vi "LabVIEW IV 2주차.vi"() -> ()   [LabVIEW 2025]
uses:
  <vilib>/Analysis/1siggen.llb/Ramp Pattern by Samples.vi
  <vilib>/Analysis/NI_AALBase.lvlib
panel:
  in  "VISA resource name 2":refnum<visa-resource-name>
  in  "Start":bool
  in  "Both forward & backward sweep":bool=TRUE
  in  "VISA resource name":refnum<visa-resource-name>="GPIB0::15::INSTR"
  in  "stop":bool
  in  "samples":i32=128
  in  "Voltage End":dbl=1.0
  in  "Voltage start":dbl
  out "XY Graph":cluster{"Y":dbl[], "Y":dbl[]}[](graph)
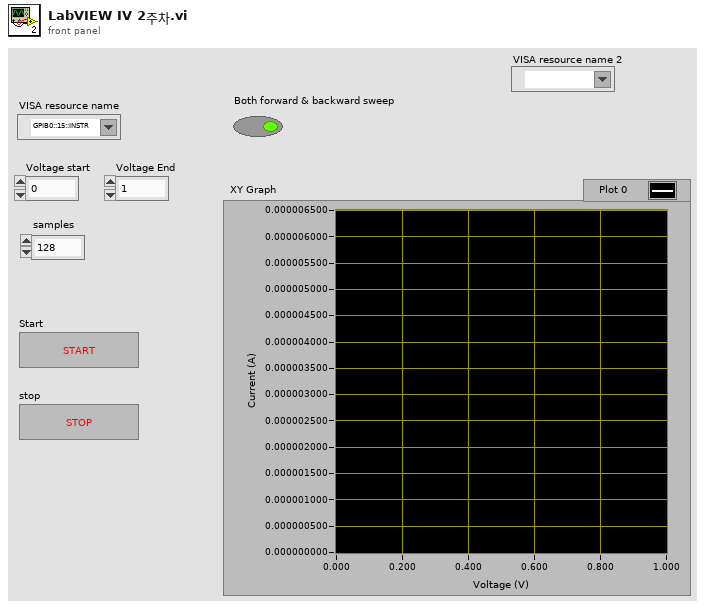
[diagram p1: front panel]
types:
  T1 = enum16{"open", "replace", "create", "open or create", "replace or create", "replace or create with confirmation"}
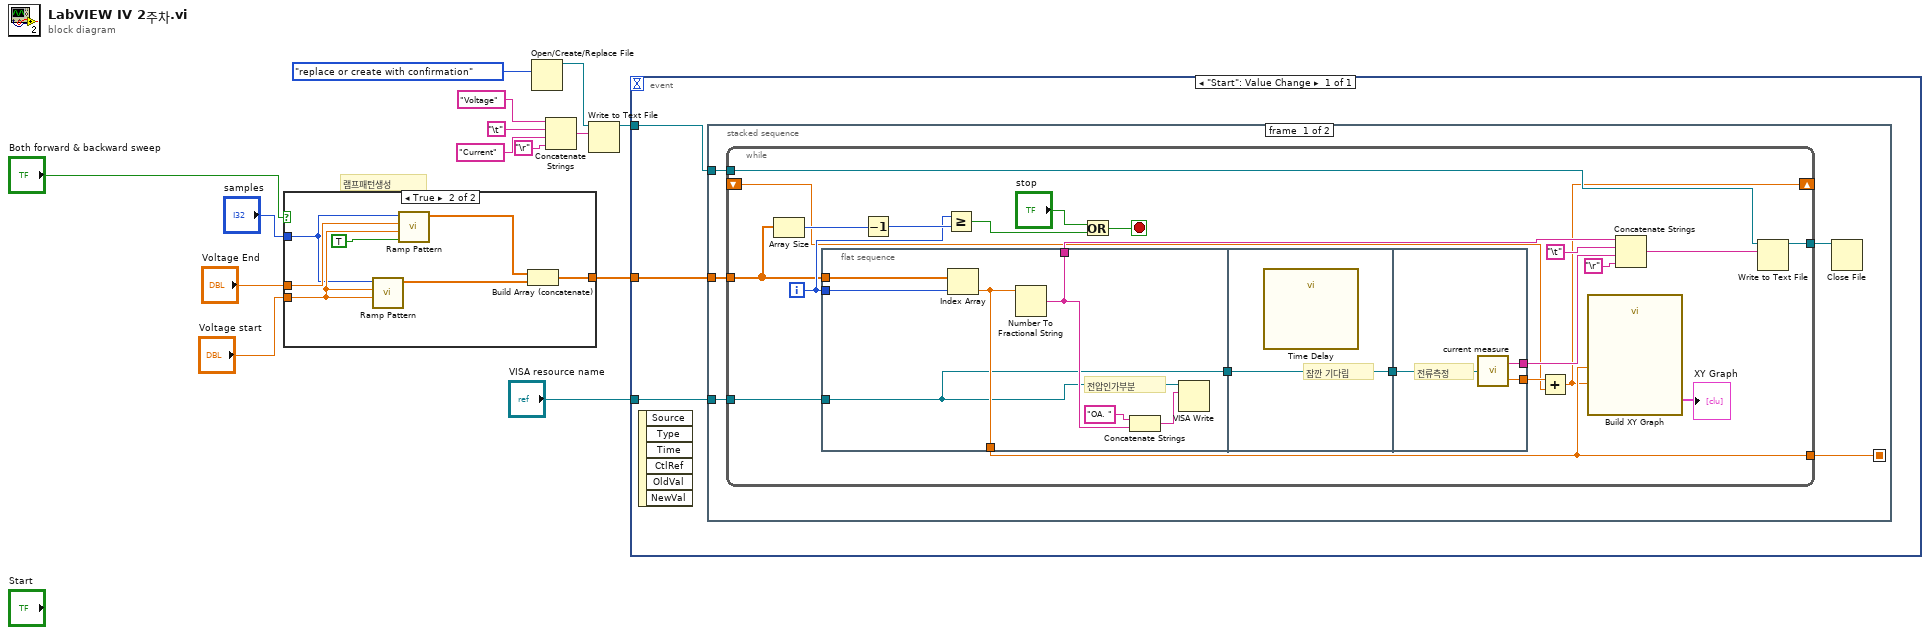
[diagram p0: block diagram]
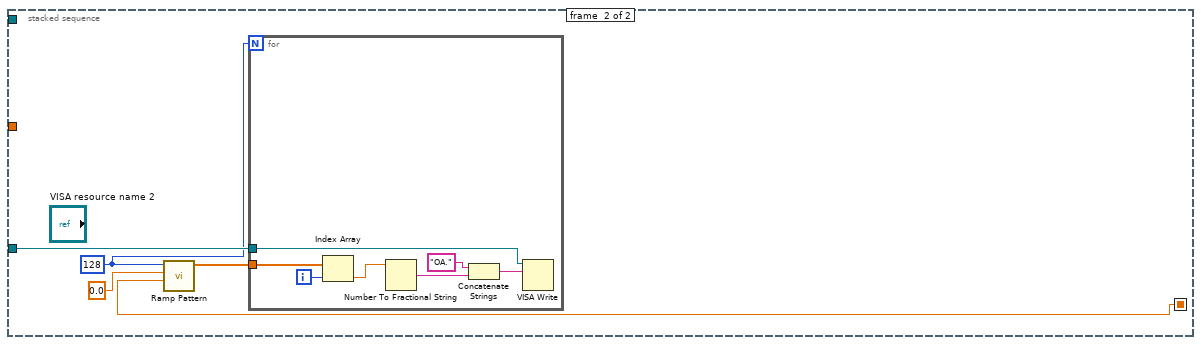
[diagram p2: hidden frame]
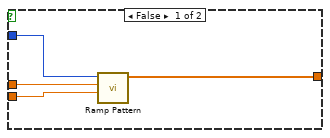
[diagram p3: hidden frame]
diagram:
  # "램프패턴생성"
  n1 = case shown="True" "Both forward & backward sweep" {
    tunnel: "Voltage start" -> [w18 w24]
    tunnel: "Voltage End" -> [w17 w25]
    tunnel: [w16 w19] -> w12
    tunnel: "samples" -> [w15 w23]
    frame False {
      n2 = call-poly <vilib>:"Ramp Pattern.vi"("start"=w18, "end"=w17, "samples"=w15) -> ("Ramp Pattern"=w16:dbl[])  [unwired: 7 in, 1 out]
    }
    frame True {
      n3 = call-poly <vilib>:"Ramp Pattern.vi"("start"=w24, "end"=w24, "samples"=w23) -> ("Ramp Pattern"=w20:dbl[])  [unwired: 7 in, 1 out]
      n4 = call-poly <vilib>:"Ramp Pattern.vi"("exclude end?"=TRUE, "start"=w24, "end"=w25, "samples"=w23) -> ("Ramp Pattern"=w21:dbl[])  [unwired: 6 in, 1 out]
      n5 = Build Array (concatenate)(w21, w20) -> (w19:dbl[])
    }
  }
  n6 = Open/Create/Replace File(operation (0:open)=T1."replace or create with confirmation") -> (refnum out=w9:refnum<file>)  [unwired: 5 in, 2 out]
  n7 = Concatenate Strings("Voltage" ("string"), "\t", "Current" ("string"), "\r") -> (w6:string)
  n8 = Write to Text File(file (use dialog)=w9, text=w6) -> (refnum out=w3:refnum<file>)  [unwired: 2 in, 2 out]
  n9 = event shown="[0] \"Start\": Value Change" {
    selector: _ -> [_]
    dyn-events: _ -> [_]
    timeout: _ -> [_]
    tunnel: w12 -> [w28]
    tunnel: w3 -> [w27]
    tunnel: "VISA resource name" -> [w26]
    event "Start": Value Change {
      n10 = event-data() -> ()  [unwired: 1 in, 6 out]
      n11 = stacked-sequence {
        seq-local: [w29 _] -> [_ w70]
        tunnel: w28 -> [w33 _]
        tunnel: w27 -> [w31 _]
        tunnel: w26 -> [w30 w68]
        frame #0 {
          n12 = while {
            tunnel: w33 -> [w40]
            tunnel: w31 -> [w50]
            tunnel: [w49] -> w32
            tunnel: w30 -> [w43]
            tunnel: [w37] -> w29
            shift-right: [w34] -> _
            shift-left: _ -> [w35]
            i -> [w51]
            stop <- w38 stop-if-true
            n13 = Array Size(array=w40) -> (size(s)=w39:i32)
            n14 = flat-sequence {
              tunnel: w40 -> [w62]
              tunnel: w51 -> [w61]
              tunnel: [w60] -> w37
              tunnel: [w57] -> w48
              tunnel: w43 -> [w56]
              tunnel: [w56] -> w41
              tunnel: [w63] -> w42
              tunnel: w41 -> [w63]
              tunnel: [w65] -> w47
              tunnel: w42 -> [w66]
              tunnel: [w64] -> w36
              frame #0 {
                # "전압인가부분"
                n15 = Index Array(array=w62, index=w61) -> (element=w60:dbl)
                n16 = Number To Fractional String(number=w60) -> (F-format string=w57:string)  [unwired: 3 in]
                n17 = Concatenate Strings("OA. " ("write buffer"), w57) -> (w59:string)
                n18 = VISA Write(VISA resource name=w56, write buffer=w59) -> ()  [unwired: 1 in, 3 out]
              }
              frame #1 {
                # "잠깐 기다림"
                n19 = call "Time Delay"() -> ()  [unwired: 11 in, 1 out]
              }
              frame #2 {
                # "전류측정"
                n20 = call "current measure.vi"("VISA Refnum in"=w66) -> ("read buffer"=w65:string, "Numeric"=w64:dbl)
              }
            }
            n21 = Decrement(x=w39) -> (x-1=w54:i32)
            n22 = Greater Or Equal?(x=w51, y=w54) -> (x >= y?=w52:bool)
            n23 = Or(x="stop", y=w52) -> (x .or. y?=w38:bool)
            n24 = Add(x=w36, y=w35) -> (x+y=w34:dbl)
            n25 = call "Build XY Graph"("Y Input"=w34, "X Input"=w37) -> ("XY Graph"=→"XY Graph":cluster{"X":dbl[], "Y":dbl[]}[])  [unwired: 8 in, 1 out]
            n26 = Concatenate Strings(w48, "\t", w47, "\r") -> (w44:string)
            n27 = Write to Text File(file (use dialog)=w50, text=w44) -> (refnum out=w49:refnum<file>)  [unwired: 2 in, 2 out]
          }
          n28 = Close File(refnum=w32) -> ()  [unwired: 1 in, 2 out]
        }
        frame #1 {
          w67 = 128 ("samples")
          n29 = call-poly <vilib>:"Ramp Pattern.vi"("start"=w70, "end"=0.0, "samples"=w67) -> ("Ramp Pattern"=w69:dbl[])  [unwired: 7 in, 1 out]
          n30 = for {
            N: w67 -> [_]
            tunnel: w69 -> [w75]
            tunnel: w68 -> [w76]
            i -> [w74]
            n31 = Index Array(array=w75, index=w74) -> (element=w73:dbl)
            n32 = Number To Fractional String(number=w73) -> (F-format string=w72:string)  [unwired: 3 in]
            n33 = Concatenate Strings("OA." ("write buffer"), w72) -> (w77:string)
            n34 = VISA Write(VISA resource name=w76, write buffer=w77) -> ()  [unwired: 1 in, 3 out]
          }
        }
      }
    }
  }
